vi "macro_TrajectoryConstraint_DiffKine.vi"   [LabVIEW 2019, in "Trajectory_Library.lvlib"]
uses:
  Trajectory_Library.lvlib
types:
  T1 = typedef "Trajectory_Library.lvlib/DIFF_DRIVE_KINEMATICS.ctl" = cluster{"TrackWidth_Meters":dbl}
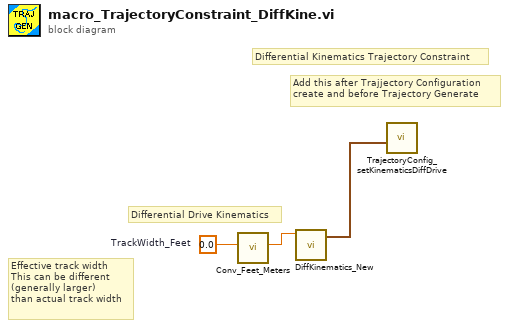
[diagram p0: block diagram]
diagram:
  w2 = 0.0  # TrackWidth_Feet
  # "Differential Kinematics Trajectory Constraint"
  # "Add this after Trajjectory Configuration\ncreate and before Trajectory Generate"
  # "Differential Drive Kinematics"
  # "Effective track width\nThis can be different\n(generally larger)\nthan actual track width"
  n1 = call "Conv_Feet_Meters.vi"("Feet"=w2) -> ("Meters"=w3:dbl)  [unwired: 10 in]
  n2 = call "DiffKinematics_New.vi"("TrackWidth_Meters"=w3) -> ("DIFF_DRIVE_KINEMATICS"=w1:T1)  [unwired: 10 in]
  n3 = call "TrajectoryConfig_setKinematicsDiffDrive.vi"("DIFF_DRIVE_KINEMATICS"=w1) -> ()  [unwired: 10 in, 1 out]
